vi "Query-save-characteristics.vi"(8 "error in":errorcluster, 11 "Storage params. ref. in":refnum<data-value>) -> (0 "error IO":errorcluster, 2 "Save characteristics?":bool, 3 "Storage params. ref.":refnum<data-value>)   [LabVIEW 2013, in "CameraVision.lvlib" / "CV-Storage.lvclass"]
doc: "This function increases the layer/iteration number by one (+1)."
uses:
  CV-Storage.lvclass
  CV-Storage.lvclass/CV-Storage.ctl
  Read Save what.vi
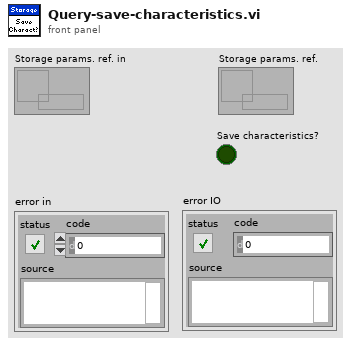
[diagram p1: front panel]
types:
  T1 = cluster{"Original":bool, "Corrected":bool, "Binary":bool, "Temperature":bool, "Characteristics":bool, "Mapping":bool, "TemperatureValues":bool}
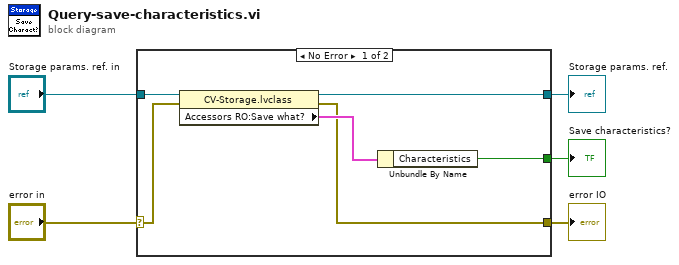
[diagram p0: block diagram]
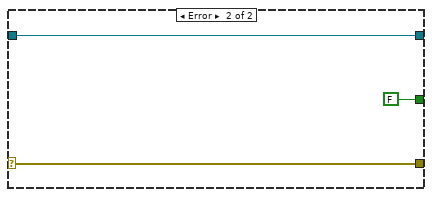
[diagram p2: hidden frame]
diagram:
  n1 = case shown="No Error" "error in" {
    selector: "error in" -> [w10 w14]
    tunnel: [w7 w14] -> w4
    tunnel: "Storage params. ref. in" -> [w11 w13]
    tunnel: [w9 w13] -> w2
    tunnel: [w6 FALSE] -> w1
    frame No Error {
      n2 = property class="CV-Storage.lvclass"(reference=w11, error in=w10) -> (reference out=w9:refnum<data-value>, error out=w7:errorcluster, "Accessors RO:Save what?"=w8:T1)
      n3 = Unbundle By Name(w8) -> ("Characteristics"=w6:bool)
    }
    frame Error {
    }
  }
  "error IO" <- w4
  "Storage params. ref." <- w2
  "Save characteristics?" <- w1
